vi "Get_Win_Pos.vi"(8 "error in (no error)":errorcluster, 11 "Win Name":string) -> (0 "error out":errorcluster, 3 "Win_Position":cluster{"x":sgl, "y":sgl})   [LabVIEW 2025]
uses:
  user32.dll
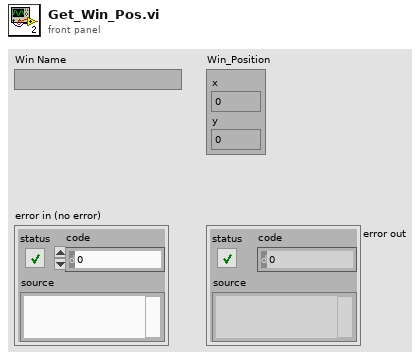
[diagram p1: front panel]
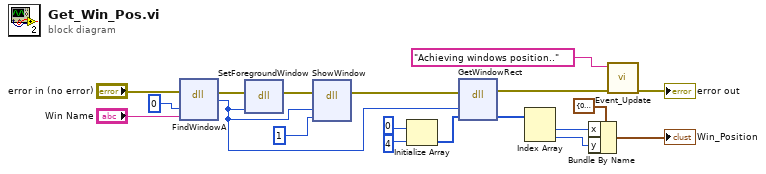
[diagram p0: block diagram]
diagram:
  n1 = dll-call lib="user32.dll" fn="FindWindowA"(error in="error in (no error)", "arg1"=0, "arg2"="Win Name") -> (error out=w10:errorcluster, "return type"=w8:i32)  [unwired: 3 in, 2 out]
  n2 = dll-call lib="user32.dll" fn="SetForegroundWindow"(error in=w10, "arg1"=w8) -> (error out=w11:errorcluster)  [unwired: 3 in, 2 out]
  n3 = dll-call lib="user32.dll" fn="ShowWindow"(error in=w11, "arg1"=w8, "arg2"=1) -> (error out=w9:errorcluster)  [unwired: 4 in, 2 out]
  n4 = Initialize Array(0, 4) -> (w16:i32[])
  n5 = dll-call lib="USER32.DLL" fn="GetWindowRect"(error in=w9, "hWnd"=w8, "RECT"=w16) -> (error out=w5:errorcluster, "RECT"=w1:i32[])  [unwired: 3 in, 2 out]
  n6 = Index Array(array=w1) -> (element #1=w14:i32, element #2=w13:i32)  [unwired: 2 in]
  n7 = Bundle By Name(cluster=cluster{"x":sgl, "y":sgl} {"x"=0.0, "y"=0.0} ("Position"), "x"=w14, "y"=w13) -> (→"Win_Position":cluster{"x":sgl, "y":sgl})
  n8 = call "Event_Update.vi"("Error In"=w5, "Event"="Achieving windows position..") -> ("Error Out"=→"error out":errorcluster)  [unwired: 9 in]
